vi "TCP Buffered Read.vi"(8 "error in (no error)":errorcluster, 9 "timeout (ms)":i32=5000, 11 "connection ID":refnum<k5>) -> (0 "error out":errorcluster, 1 "Final packet":bool, 2 "data string":string, 3 "connection ID 2":refnum<k5>)   [LabVIEW 2015]
panel:
  out "Numeric":i32
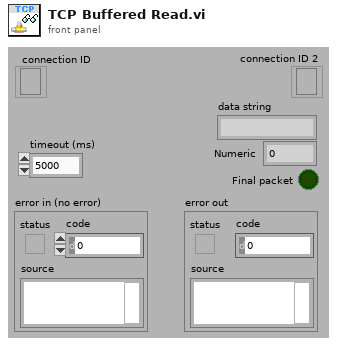
[diagram p1: front panel]
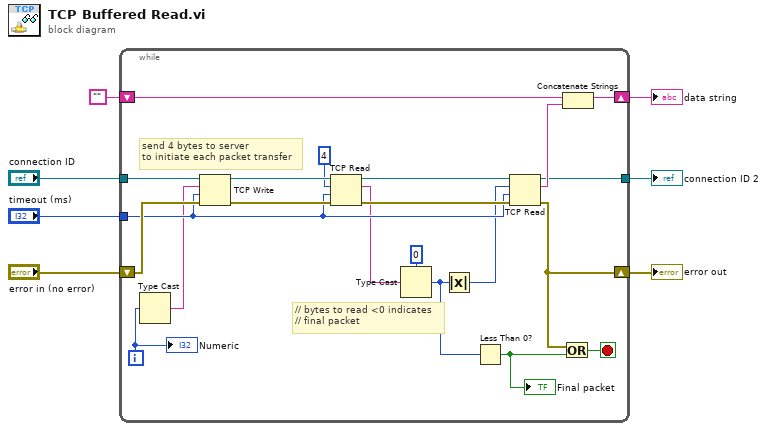
[diagram p0: block diagram]
diagram:
  n1 = while {
    tunnel: "connection ID" -> [w26]
    shift-right: [w8] -> w7
    shift-left: "error in (no error)" -> [w25]
    tunnel: "timeout (ms)" -> [w22]
    shift-right: [w21] -> w2
    shift-left: "" -> [w20]
    tunnel: [w10] -> w1
    i -> [w19]
    stop <- w9 stop-if-true
    # "// bytes to read <0 indicates\n// final packet"
    # "send 4 bytes to server \nto initiate each packet transfer"
    n2 = Type Cast(x=w19) -> (*(type *) &x=w18:string)  [unwired: 1 in]
    n3 = TCP Write(connection ID=w26, data in=w18, error in (no error)=w25, 9:w22) -> (connection ID out=w24:refnum<k5>, error out=w23:errorcluster)  [unwired: 1 out]
    n4 = TCP Read(connection ID=w24, bytes to read=4, error in (no error)=w23, 9:w22) -> (connection ID out=w28:refnum<k5>, data out=w16:string, error out=w27:errorcluster)  [unwired: 1 in]
    n5 = Type Cast(type=0, x=w16) -> (*(type *) &x=w13:i32)
    n6 = Absolute Value(x=w13) -> (abs(x)=w14:i32)
    n7 = Less Than 0?(x=w13) -> (x < 0?=w11:bool)
    "Final packet" <- w11
    n8 = TCP Read(connection ID=w28, bytes to read=w14, error in (no error)=w27, 9:w22) -> (connection ID out=w10:refnum<k5>, data out=w12:string, error out=w8:errorcluster)  [unwired: 1 in]
    n9 = Or(x=w8, y=w11) -> (x .or. y?=w9:bool)
    n10 = Concatenate Strings(w20, w12) -> (w21:string)
    "Numeric" <- w19
  }
  "error out" <- w7
  "data string" <- w2
  "connection ID 2" <- w1
